vi "RSZVB Trace Import Data.vi"(8 "error in (no error)":errorcluster {"code" format="%.0x"}, 9 "File Name (Trc1.s1p)":string="Trc1.s1p", 10 "Trace Name (Trc1)":string="Trc1", 11 "VISA session":refnum<visa-resource-name>) -> (0 "error out":errorcluster {"code" format="%.0x"}, 3 "dup VISA session":refnum<visa-resource-name>)   [LabVIEW 2011]
doc: "This VI loads trace data from a specified trace file and assigns it to a trace with a specified name.\n\nNote(s):\n\nTraces are created using the CALCulte<Ch>:PARameter:SDEFine... command.\n\nRemote-control command(s):\nMMEMory:LOAD:TRACe '<trc_name>','<file_name>'[,'<parameter_name>']"
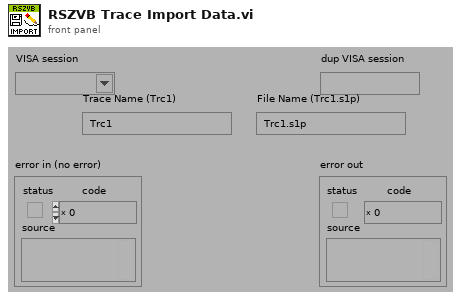
[diagram p1: front panel]
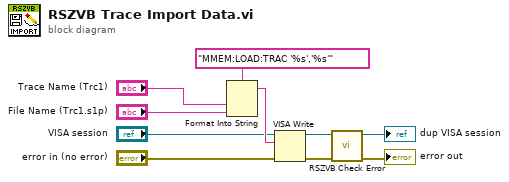
[diagram p0: block diagram]
diagram:
  n1 = Format Into String(format string="MMEM:LOAD:TRAC '%s','%s'", "Trace Name (Trc1)", "File Name (Trc1.s1p)") -> (resulting string=w7:string)  [unwired: 2 in, 1 out]
  n2 = VISA Write(VISA resource name="VISA session", write buffer=w7, error in (no error)="error in (no error)") -> (VISA resource name out=w8:refnum<visa-resource-name>, error out=w9:errorcluster)  [unwired: 1 out]
  n3 = call "RSZVB Check Error.vi"("error in (no error)"=w9, "VISA session"=w8) -> ("error out"=→"error out":errorcluster, "dup VISA session"=→"dup VISA session":refnum<visa-resource-name>)  [unwired: 8 in]
